vi "Port to Transducer.vi"(11 "Numeric":i32) -> (2 "Found?":bool, 3 "Sensor":T1)   [LabVIEW 2015]
uses:
  Sensor Enum.ctl
  Sensor Port Mapping Global Action.ctl
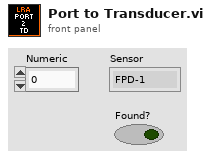
[diagram p1: front panel]
types:
  T1 = typedef "Sensor Enum.ctl" = enum16{"FPD-1", "OPD-1", "FPD-2", "OPD-2"}
  T2 = typedef "Sensor Port Mapping Global Action.ctl" = enum16{"Get", "Set"}
  T3 = typedef "Sensor Port Mapping.ctl" = cluster{"Sensor":T1, "Thermocouple?":bool, "Port":u32}
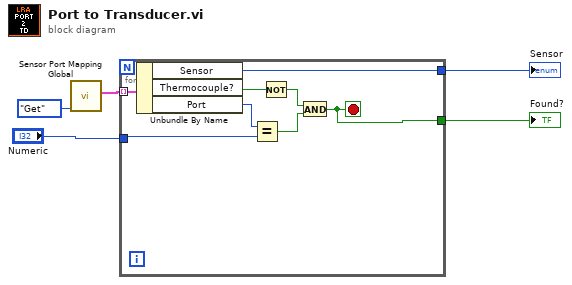
[diagram p0: block diagram]
diagram:
  n1 = call "Sensor Port Mapping Global.vi"("Action"=Sensor_Port_Mapping_Global_Action."Get") -> ("Mapping List"=w2:T3[])  [unwired: 10 in]
  n2 = for {
    tunnel: w2 -> [w13] mode=indexing
    tunnel: "Numeric" -> [w11]
    tunnel: [w7] -> w4
    tunnel: [w6] -> w5
    stop <- w6 stop-if-true
    n3 = Unbundle By Name(w13) -> ("Sensor"=w7:T1, "Thermocouple?"=w10:bool, "Port"=w12:u32)
    n4 = Equal?(x=w12, y=w11) -> (x = y?=w8:bool)
    n5 = Not(x=w10) -> (.not. x?=w9:bool)
    n6 = And(x=w9, y=w8) -> (x .and. y?=w6:bool)
  }
  "Found?" <- w5
  "Sensor" <- w4
